vi "Pi-Drive - Momentum (SubVI).vi"(9 "True - Momentum On\nFalse - Momentum Off":bool, 10 "Momentum Gain":dbl, 11 "Turn in":dbl) -> (3 "Turn out":dbl)   [LabVIEW 2019]
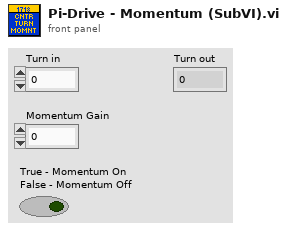
[diagram p1: front panel]
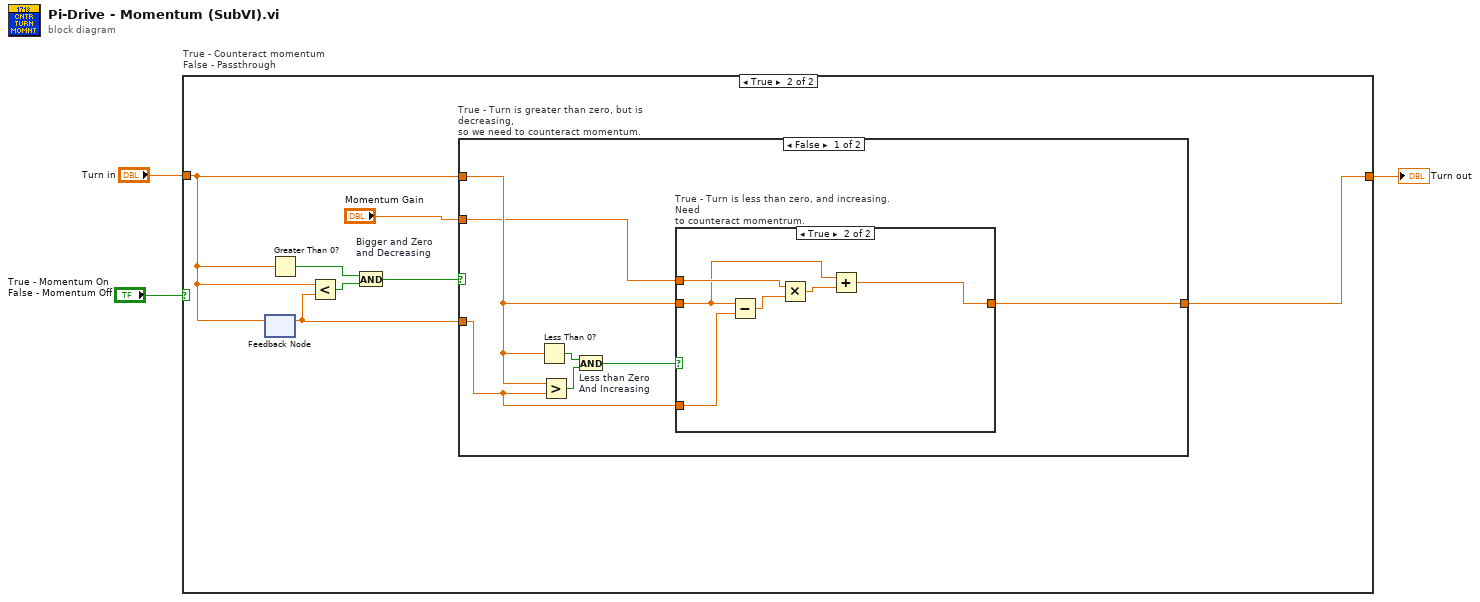
[diagram p0: block diagram]
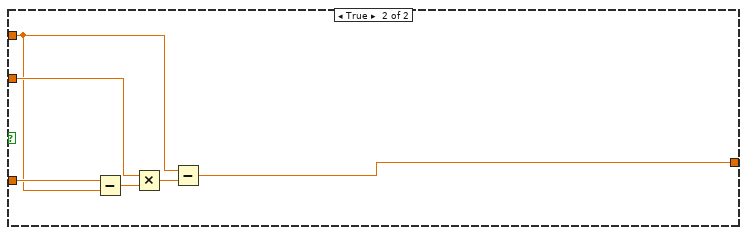
[diagram p4: hidden frame]
diagram:
  n1 = case "True - Counteract momentum\nFalse - Passthrough" shown="True" "True - Momentum On\nFalse - Momentum Off" {
    tunnel: "Turn in" -> [w4 w6]
    tunnel: [w4 w5] -> w2
    frame False {
    }
    frame True {
      n2 = feedback #1() -> (w7:dbl)  [unwired: 1 in]
      n3 = feedback-in #1(w6) -> ()
      n4 = Greater Than 0?(x=w6) -> (x > 0?=w10:bool)
      n5 = Less?(x=w6, y=w7) -> (x < y?=w11:bool)
      n6 = And "Bigger and Zero\nand Decreasing"(x=w10, y=w11) -> (x .and. y?=w8:bool)
      n7 = case "True - Turn is greater than zero, but is decreasing,\nso we need to counteract momentum." shown="False" w8 {
        tunnel: "Momentum Gain" -> [w13 w29]
        tunnel: w6 -> [w14 w27]
        tunnel: w7 -> [w15 w28]
        tunnel: [w12 w26] -> w5
        frame False {
          n8 = Less Than 0?(x=w14) -> (x < 0?=w17:bool)
          n9 = Greater?(x=w14, y=w15) -> (0:w16:bool)
          n10 = And "Less than Zero\nAnd Increasing"(x=w17, y=w16) -> (x .and. y?=w18:bool)
          n11 = case "True - Turn is less than zero, and increasing.  Need\nto counteract momentrum." shown="True" w18 {
            tunnel: w15 -> [_ w25]
            tunnel: w14 -> [w19 w21]
            tunnel: w13 -> [_ w23]
            tunnel: [w19 w20] -> w12
            frame False {
            }
            frame True {
              n12 = Subtract(x=w21, y=w25) -> (x-y=w24:dbl)
              n13 = Multiply(x=w23, y=w24) -> (x*y=w22:dbl)
              n14 = Add(x=w21, y=w22) -> (x+y=w20:dbl)
            }
          }
        }
        frame True {
          n15 = Subtract(x=w28, y=w27) -> (x-y=w31:dbl)
          n16 = Multiply(x=w29, y=w31) -> (x*y=w30:dbl)
          n17 = Subtract(x=w27, y=w30) -> (x-y=w26:dbl)
        }
      }
    }
  }
  "Turn out" <- w2
